vi "VMI_make_x.vi"(2 "Graph X":i32[](array[numeric]), 3 "Types to acquire in":bool[](array[boolean])) -> (0 "CompiledX":i32[][](array[numeric]))   [LabVIEW 2019]
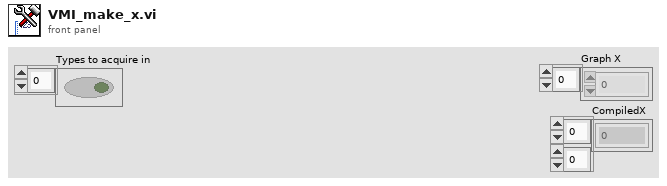
[diagram p1: front panel]
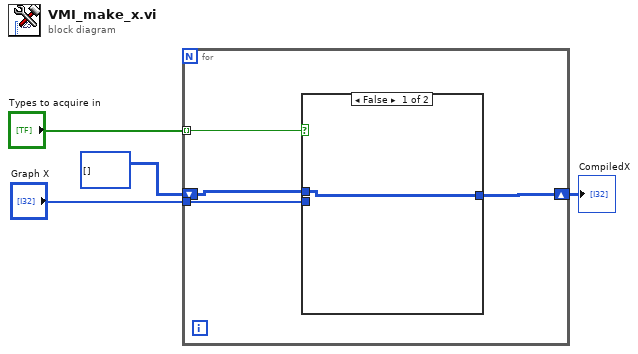
[diagram p0: block diagram]
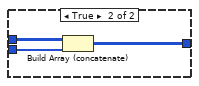
[diagram p2: hidden frame]
diagram:
  n1 = for {
    tunnel: "Types to acquire in" -> [w8] mode=indexing
    tunnel: "Graph X" -> [w7]
    shift-right: [w6] -> w1
    shift-left: i32[][] [] -> [w5]
    n2 = case shown="False" w8 {
      tunnel: w7 -> [_ w12]
      tunnel: [w9 w11] -> w6
      tunnel: w5 -> [w9 w10]
      frame False {
      }
      frame True {
        n3 = Build Array (concatenate)(w10, w12) -> (w11:i32[][])
      }
    }
  }
  "CompiledX" <- w1
